vi "Command Lift.vi"(7 "Startup":bool, 9 "Timeout":u32=5, 10 "Set Position":T1=enum."Load") -> (3 "Lift Out":dbl, 4 "Reinit":bool, 6 "Completed":bool)   [LabVIEW 2017]
uses:
  Lift/Lift Enum States.ctl
  Lift/Lift Globals.vi
panel:
  in  "Lift Allowable Error Down":dbl=1000.0
  out "Current Error":dbl
  in  "kP Max Down":dbl=-1.0
  in  "kP Max Up":dbl=1.0
  in  "Lift Allowable Error Up":dbl=1000.0
  in  "kP Down":dbl=4.18e-05
  in  "kP Up":dbl=0.00017
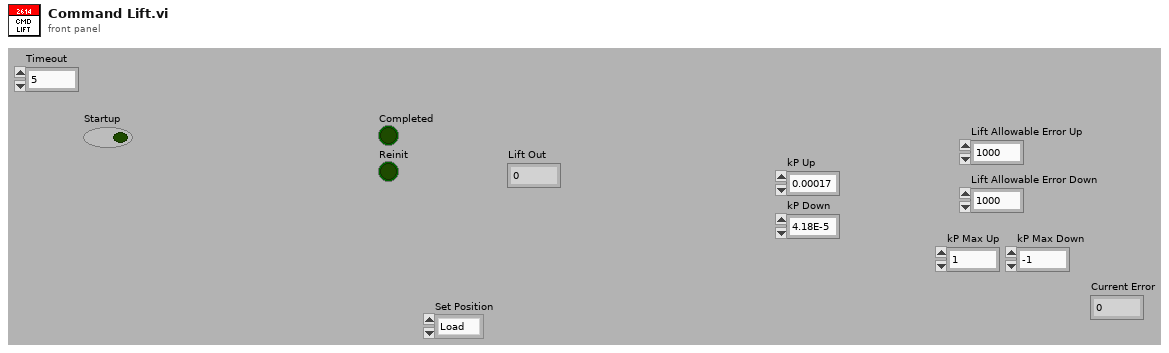
[diagram p1: front panel]
types:
  T1 = typedef "Lift Enum States.ctl" = enum16{"Climb", "Load", "Portal", "Switch", "Scale High", "Scale Mid", "Scale Low", "Exchange", "Stow", "Current Position"}
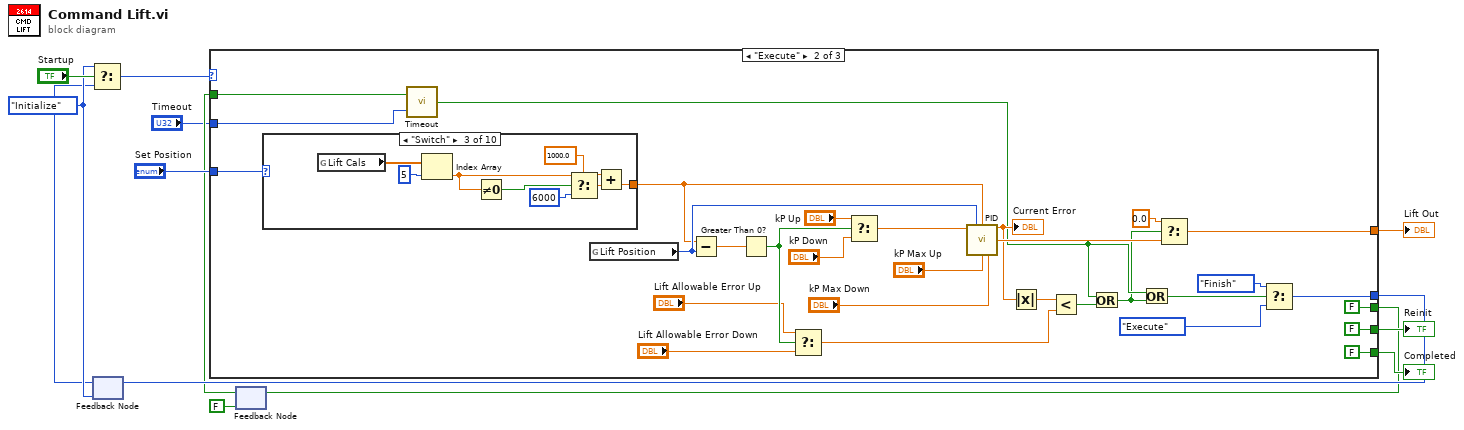
[diagram p0: block diagram]
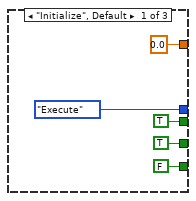
[diagram p2: hidden frame]
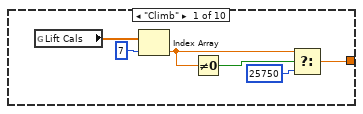
[diagram p3: hidden frame]
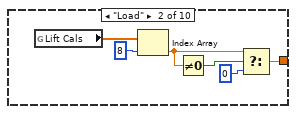
[diagram p4: hidden frame]
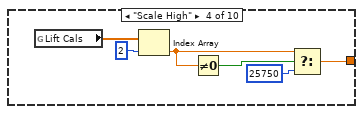
[diagram p5: hidden frame]
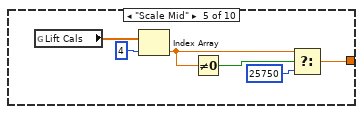
[diagram p6: hidden frame]
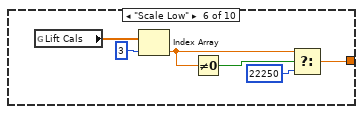
[diagram p7: hidden frame]
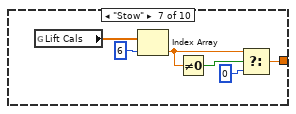
[diagram p8: hidden frame]
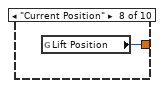
[diagram p9: hidden frame]
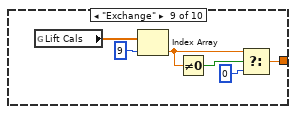
[diagram p10: hidden frame]
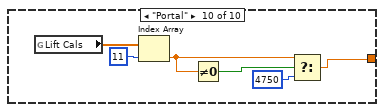
[diagram p11: hidden frame]
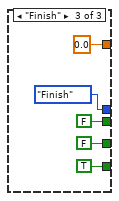
[diagram p12: hidden frame]
diagram:
  w11 = enum16{"Initialize", "Execute", "Finish"}."Initialize"
  n1 = feedback #1(w11) -> (w7:enum16{"Initialize", "Execute", "Finish"})
  n2 = Select(t=w11, s="Startup", f=w7) -> (s? t:f=w12:enum16{"Initialize", "Execute", "Finish"})
  n3 = feedback #2(FALSE) -> (w3:bool)
  n4 = case shown="\"Execute\"" w12 {
    tunnel: [FALSE FALSE TRUE] -> w10
    tunnel: [TRUE FALSE FALSE] -> w9
    tunnel: [enum16{"Initialize", "Execute", "Finish"}."Execute" w44 enum16{"Initialize", "Execute", "Finish"}."Finish"] -> w8
    tunnel: [0.0 ("Right Wheel Velocity") w21 0.0] -> w6
    tunnel: "Set Position" -> [_ w40 _]
    tunnel: [TRUE FALSE FALSE] -> w4
    tunnel: w3 -> [_ w43 _]
    tunnel: "Timeout" -> [_ w42 _]
    frame "Initialize", Default {
    }
    frame "Execute" {
      n5 = case shown="\"Switch\"" w40 {
        tunnel: [w49 w56 w62 w69 w75 w81 w89 w93 w94 w100] -> w20
        frame "Climb" {
          n6 = global read "Lift Globals.vi" "Lift Cals"() -> (w54:dbl[])
          n7 = Index Array(array=w54, index=7) -> (element=w51:dbl)
          n8 = Not Equal To 0?(x=w51) -> (x != 0?=w52:bool)
          n9 = Select(t=w51, s=w52, f=25750 ("Lift Position")) -> (s? t:f=w49:dbl)
        }
        frame "Load" {
          n10 = global read "Lift Globals.vi" "Lift Cals"() -> (w60:dbl[])
          n11 = Index Array(array=w60, index=8) -> (element=w57:dbl)
          n12 = Not Equal To 0?(x=w57) -> (x != 0?=w58:bool)
          n13 = Select(t=w57, s=w58, f=0 ("Lift Position")) -> (s? t:f=w56:dbl)
        }
        frame "Switch" {
          n14 = global read "Lift Globals.vi" "Lift Cals"() -> (w68:dbl[])
          n15 = Index Array(array=w68, index=5) -> (element=w64:dbl)
          n16 = Not Equal To 0?(x=w64) -> (x != 0?=w66:bool)
          n17 = Select(t=w64, s=w66, f=6000 ("Lift Position")) -> (s? t:f=w63:dbl)
          n18 = Add(x=1000.0, y=w63) -> (x+y=w62:dbl)
        }
        frame "Scale High" {
          n19 = global read "Lift Globals.vi" "Lift Cals"() -> (w74:dbl[])
          n20 = Index Array(array=w74, index=2) -> (element=w70:dbl)
          n21 = Not Equal To 0?(x=w70) -> (x != 0?=w72:bool)
          n22 = Select(t=w70, s=w72, f=25750 ("Lift Position")) -> (s? t:f=w69:dbl)
        }
        frame "Scale Mid" {
          n23 = global read "Lift Globals.vi" "Lift Cals"() -> (w80:dbl[])
          n24 = Index Array(array=w80, index=4) -> (element=w76:dbl)
          n25 = Not Equal To 0?(x=w76) -> (x != 0?=w78:bool)
          n26 = Select(t=w76, s=w78, f=25750 ("Lift Position")) -> (s? t:f=w75:dbl)
        }
        frame "Scale Low" {
          n27 = global read "Lift Globals.vi" "Lift Cals"() -> (w86:dbl[])
          n28 = Index Array(array=w86, index=3) -> (element=w82:dbl)
          n29 = Not Equal To 0?(x=w82) -> (x != 0?=w84:bool)
          n30 = Select(t=w82, s=w84, f=22250 ("Lift Position")) -> (s? t:f=w81:dbl)
        }
        frame "Stow" {
          n31 = global read "Lift Globals.vi" "Lift Cals"() -> (w92:dbl[])
          n32 = Index Array(array=w92, index=6) -> (element=w88:dbl)
          n33 = Not Equal To 0?(x=w88) -> (x != 0?=w90:bool)
          n34 = Select(t=w88, s=w90, f=0 ("Lift Position")) -> (s? t:f=w89:dbl)
        }
        frame "Current Position" {
          n35 = global read "Lift Globals.vi" "Lift Position"() -> (w93:i32)
        }
        frame "Exchange" {
          n36 = global read "Lift Globals.vi" "Lift Cals"() -> (w99:dbl[])
          n37 = Index Array(array=w99, index=9) -> (element=w95:dbl)
          n38 = Not Equal To 0?(x=w95) -> (x != 0?=w97:bool)
          n39 = Select(t=w95, s=w97, f=0 ("Lift Position")) -> (s? t:f=w94:dbl)
        }
        frame "Portal" {
          n40 = global read "Lift Globals.vi" "Lift Cals"() -> (w105:dbl[])
          n41 = Index Array(array=w105, index=11) -> (element=w101:dbl)
          n42 = Not Equal To 0?(x=w101) -> (x != 0?=w103:bool)
          n43 = Select(t=w101, s=w103, f=4750 ("Lift Position")) -> (s? t:f=w100:dbl)
        }
      }
      n44 = call "Timeout.vi"("Timeout"=w42, "Initialize"=w43) -> ("Timed Out?"=w22:bool)
      n45 = global read "Lift Globals.vi" "Lift Position"() -> (w31:i32)
      n46 = Subtract(x=w20, y=w31) -> (x-y=w32:dbl)
      n47 = Greater Than 0?(x=w32) -> (x > 0?=w27:bool)
      n48 = Select(t="Lift Allowable Error Up", s=w27, f="Lift Allowable Error Down") -> (s? t:f=w26:dbl)
      n49 = Select(t="kP Up", s=w27, f="kP Down") -> (s? t:f=w35:dbl)
      n50 = call "PID.vi"("Kp"=w35, "Process Variable"=w31, "Goal"=w20, "Max Ouput"="kP Max Up", "Min Output"="kP Max Down") -> ("Current Error"=w28:dbl, "Command"=w37:dbl)  [unwired: 8 in, 1 out]
      "Current Error" <- w28
      n51 = Absolute Value(x=w28) -> (abs(x)=w36:dbl)
      n52 = Less?(x=w36, y=w26) -> (x < y?=w23:bool)
      n53 = Or(x=w22, y=w23) -> (x .or. y?=w19:bool)
      n54 = Or(x=w22, y=w19) -> (x .or. y?=w39:bool)
      n55 = Select(t=0.0, s=w19, f=w37) -> (s? t:f=w21:dbl)
      n56 = Select(t=enum16{"Initialize", "Execute", "Finish"}."Finish", s=w39, f=enum16{"Initialize", "Execute", "Finish"}."Execute") -> (s? t:f=w44:enum16{"Initialize", "Execute", "Finish"})
    }
    frame "Finish" {
    }
  }
  "Completed" <- w10
  "Reinit" <- w9
  "Lift Out" <- w6
  n57 = feedback-in #1(w8) -> ()
  n58 = feedback-in #2(w4) -> ()
